vi "Convert Piccolo Hist Dataset.vi"() -> ()   [LabVIEW 2021, in "Piccolo.lvlib"]
uses:
  <vilib>/Utility/error.llb/Error Cluster From Error Code.vi
  <vilib>/ErrorRing/Error Ring.xnode
  Piccolo.lvlib
panel:
  in  "File Name Root":string
  in  "Destination Folder Path":path
  out "cancelled":bool
  out "Error Out":errorcluster
  in  "Error In":errorcluster
  in  "Source File Path":path
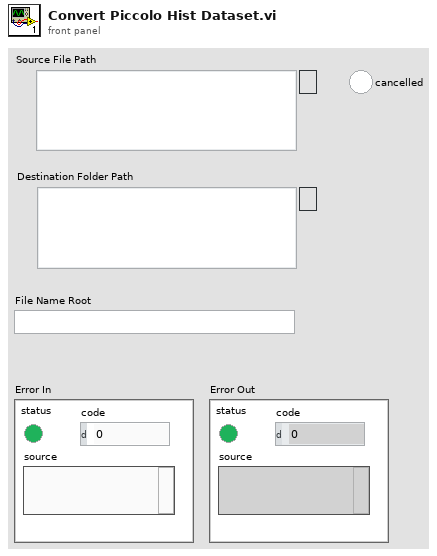
[diagram p1: front panel]
types:
  T1 = enum16{"big-endian, network order", "native, host order", "little-endian"}
  T2 = enum16{"open", "replace", "create", "open or create", "replace or create", "replace or create with confirmation"}
  T3 = typedef "imagedata.ctl" = cluster{"image type":i32, "image depth":i32, "image":u8[], "mask":u8[], "colors":u32[], "Rectangle":cluster{"left":i16, "top":i16, "right":i16, "bottom":i16}}
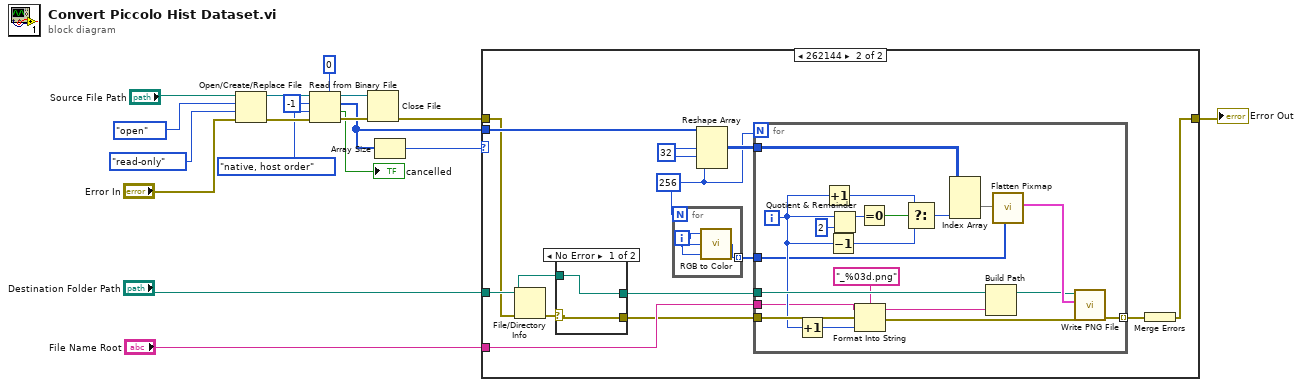
[diagram p0: block diagram]
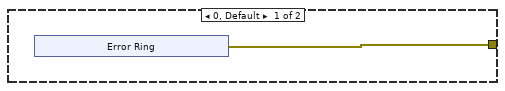
[diagram p2: hidden frame]
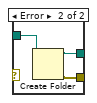
[diagram p3: hidden frame]
diagram:
  n1 = Open/Create/Replace File(file path (use dialog)="Source File Path", error in="Error In", operation (0:open)=T2."open", access (0:read/write)=enum16{"read/write", "read-only", "write-only"}."read-only") -> (refnum out=w14:refnum<file>, error out=w13:errorcluster)  [unwired: 2 in, 1 out]
  n2 = Read from Binary File(5:u16 0, 8:w13, 9:T1."native, host order" ("byte order (0:big-endian, network order)"), 10:-1 ("count (1)"), 11:w14) -> (0:w10:errorcluster, 1:→"cancelled":bool, 2:w6:u16[], 3:w11:refnum<file>)  [unwired: 1 in]
  n3 = Close File(refnum=w11, error in=w10) -> (error out=w5:errorcluster)  [unwired: 1 out]
  n4 = Array Size(array=w6) -> (size(s)=w7:i32)
  n5 = case shown="262144" w7 {
    tunnel: w6 -> [_ w36]
    tunnel: w5 -> [_ w25]
    tunnel: [w19 w32] -> w4
    tunnel: "Destination Folder Path" -> [_ w27]
    tunnel: "File Name Root" -> [_ w31]
    frame 0, Default {
      n6 = xnode "Error Ring"() -> ("error out"=w19:errorcluster)
    }
    frame 262144 {
      w34 = 32 ("dimension size")
      w30 = 256 ("dimension size")
      n7 = File/Directory Info(path=w27, error in=w25) -> (error out=w28:errorcluster)  [unwired: 6 out]
      n8 = case shown="No Error" w28 {
        selector: w28 -> [w37 _]
        tunnel: w27 -> [w38 w41]
        tunnel: [w37 w40] -> w26
        tunnel: [w38 w39] -> w24
        frame No Error {
        }
        frame Error {
          n9 = Create Folder(path (use dialog)=w41) -> (created path=w39:path, error out=w40:errorcluster)  [unwired: 2 in, 1 out]
        }
      }
      n10 = for {
        N: w30 -> [_]
        tunnel: [w42] -> w29 mode=indexing
        i -> [w43]
        n11 = call <vilib>:"RGB to Color.vi"("B"=w43, "G"=w43, "R"=w43) -> ("Color"=w42:u32)
      }
      n12 = Reshape Array(w36, w34, w34, w30) -> (w35:u16[][][])
      n13 = for {
        N: w30 -> [_]
        tunnel: w35 -> [w63]
        tunnel: w24 -> [w52]
        tunnel: w26 -> [w51]
        tunnel: [w54] -> w33 mode=indexing
        tunnel: w31 -> [w45]
        tunnel: w29 -> [w44]
        i -> [w47]
        n14 = Increment(x=w47) -> (x+1=w46:i32)
        n15 = Increment(x=w47) -> (x+1=w58:i32)
        n16 = Decrement(x=w47) -> (x-1=w57:i32)
        n17 = Quotient & Remainder(x=w47, y=u8 2) -> (x-y*floor(x/y)=w61:i32)  [unwired: 1 out]
        n18 = Format Into String(format string="_%03d.png", initial string=w45, error in=w51, w46) -> (resulting string=w49:string, error out=w50:errorcluster)
        n19 = Equal To 0?(x=w61) -> (x = 0?=w60:bool)
        n20 = Select(t=w58, s=w60, f=w57) -> (s? t:f=w59:i32)
        n21 = Index Array(array=w63, index (dim 2)=w59) -> (element=w56:u16[][])  [unwired: 2 in]
        n22 = Build Path(base path=w52, name or relative path=w49) -> (appended path=w53:path)
        n23 = call <vilib>:"Flatten Pixmap.vi"("colors"=w44, "8-bit pixmap"=w56) -> ("image data"=w55:T3)  [unwired: 9 in]
        n24 = call <vilib>:"Write PNG File.vi"("error in (no error)"=w50, "image data"=w55, "path to PNG file"=w53) -> ("error out"=w54:errorcluster)  [unwired: 7 in, 1 out]
      }
      n25 = Merge Errors(w33) -> (w32:errorcluster)
    }
  }
  "Error Out" <- w4
